vi "Read Banking Transactions.vi"(8 "error in (no error)":errorcluster) -> (0 "error out":errorcluster, 3 "CSV Transactions":refnum<class "Banking Record.lvclass">[](array[class]))   [LabVIEW 2018]
uses:
  classes/Banking Record/Banking Record.lvclass
  <vilib>/Utility/sysdir.llb/System Directory Type.ctl
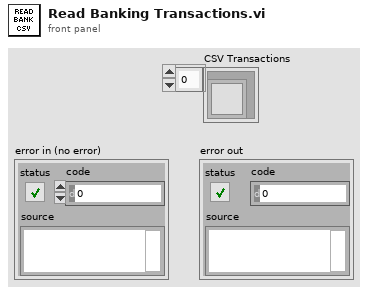
[diagram p1: front panel]
types:
  T1 = typedef "System Directory Type.ctl" = i32
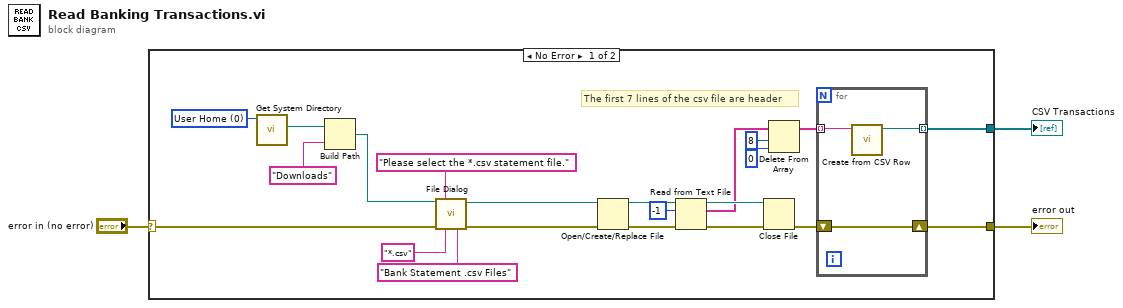
[diagram p0: block diagram]
diagram:
  n1 = case shown="No Error" "error in (no error)" {
    selector: "error in (no error)" -> [w7 w29]
    tunnel: [w4 w29] -> w3
    tunnel: [w6 _] -> w1
    frame No Error {
      w11 = T1 0 items=["User Home"=0, "User Desktop"=1, "User Documents"=2, "User Application Data"=3, "User Preferences"=4, "User Temporary"=5, "Public Documents"=6, "Public Application Data"=7, "Public Preferences"=8, "Public Cache"=13, "System Core Libraries"=9, "System Installed Libraries"=10, "Application Files"=11, "Boot Volume Root"=12] ("system directory type")
      # "The first 7 lines of the csv file are header"
      n2 = call <vilib>:"Get System Directory.vi"("system directory type"=w11) -> ("system directory"=w10:path)  [unwired: 10 in]
      n3 = Build Path(base path=w10, name or relative path="Downloads") -> (appended path=w8:path)
      n4 = call "File Dialog"("start path"=w8, "prompt"="Please select the *.csv statement file.", "error in"=w7, "pattern (all files)"="*.csv", "pattern label"="Bank Statement .csv Files") -> ("selected path"=w13:path, "error out"=w12:errorcluster)  [unwired: 2 in, 7 out]
      n5 = Open/Create/Replace File(file path (use dialog)=w13, error in=w12) -> (refnum out=w22:refnum<file>, error out=w21:errorcluster)  [unwired: 5 out]
      n6 = Read from Text File(file (use dialog)=w22, count=-1, error in=w21) -> (refnum out=w19:refnum<file>, text=w17:string[], error out=w20:errorcluster)  [unwired: 2 out]
      n7 = Close File(refnum=w19, error in=w20) -> (error out=w5:errorcluster)  [unwired: 1 out]
      n8 = Delete From Array(array=w17, length=8, index=0) -> (array with subset deleted=w14:string[])  [unwired: 1 out]
      n9 = for {
        tunnel: w14 -> [w27] mode=indexing
        tunnel: [w28] -> w6 mode=indexing
        shift-right: [w26] -> w4
        shift-left: w5 -> [w26]
        n10 = call "Create from CSV Row.vi"("CSV Row"=w27) -> ("Banking Record"=w28:refnum<class "Banking Record.lvclass">)  [unwired: 9 in, 1 out]
      }
    }
    frame Error {
    }
  }
  "error out" <- w3
  "CSV Transactions" <- w1
